vi "Save.vi"(8 "error in (no error)":errorcluster, 11 "Item in":refnum<class "Item.lvclass">) -> (0 "error out":errorcluster, 3 "Item out":refnum<class "Item.lvclass">)   [LabVIEW 2020, in "Code Cleanup.lvlib" / "Item.lvclass"]
uses:
  Item.lvclass
  Item.lvclass/Item.ctl
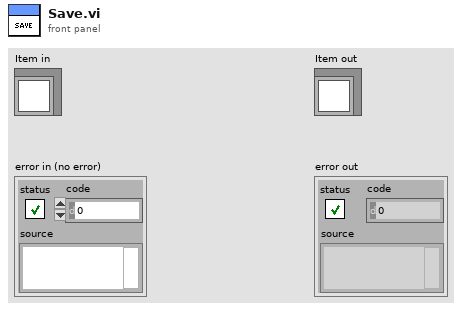
[diagram p1: front panel]
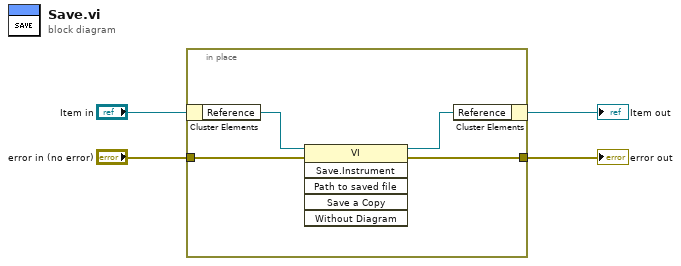
[diagram p0: block diagram]
diagram:
  n1 = in-place {
    in-place-border: "error in (no error)" -> [w7]
    in-place-border: [w5] -> w2
    n2 = in-place-cluster #1("Item in") -> ("Reference"=w8:refnum<vi>)
    n3 = invoke class="VI" method="Save.Instrument"(reference=w8, error in=w7) -> (reference out=w6:refnum<vi>, error out=w5:errorcluster)  [unwired: 4 in, 4 out]
    n4 = in-place-cluster #1("Reference"=w6) -> (→"Item out":refnum<class "Item.lvclass">)
  }
  "error out" <- w2
